vi "Simulation Lab -data type - B220061.vi"() -> ()   [LabVIEW 2020]
panel:
  out "String 2":string
  out "Meter":dbl(knob) scale=0.0..10.0
  out "Gauge":dbl(knob) scale=0.0..10.0
  in  "String":string
  out "Boolean 2":bool
  in  "Boolean":bool
  out "Numeric 2":dbl
  in  "Numeric":dbl
  in  "Slide":dbl(slide) scale=0.0..10.0
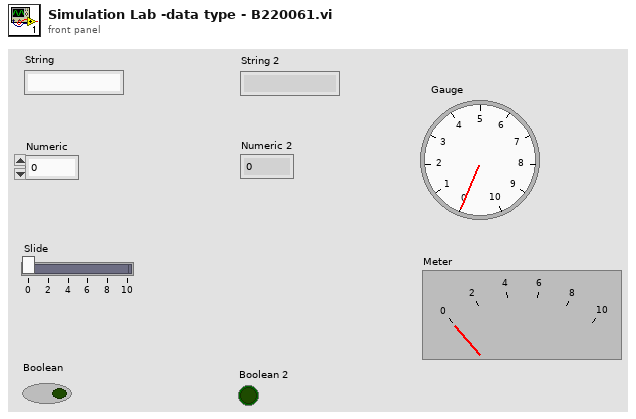
[diagram p1: front panel]
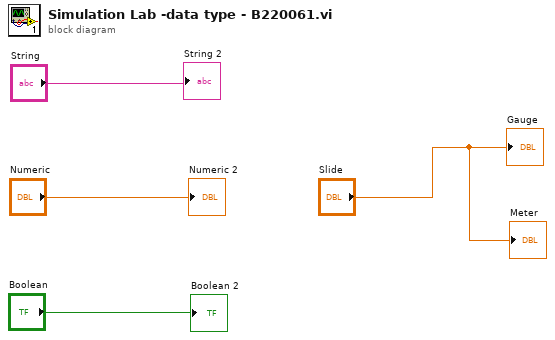
[diagram p0: block diagram]
diagram:
  "Numeric 2" <- "Numeric"
  "Boolean 2" <- "Boolean"
  "Gauge" <- "Slide"
  "Meter" <- "Slide"
  "String 2" <- "String"
